vi "BG Selection List get.vi"(0 "QD Launch VI Ref":refnum<vi>, 11 "error in (no error)":errorcluster) -> (4 "QD Launch VI Ref out":refnum<vi>, 8 "Selection List[]":refnum<vi>[](array[refnum]), 15 "error out":errorcluster)   [LabVIEW 2020, in "ColourUpStructures.lvlib"]
doc: "From QuickDrop Lunched VI reference extract All Selected GObject on Block Diagram"
uses:
  ColourUpStructures.lvlib
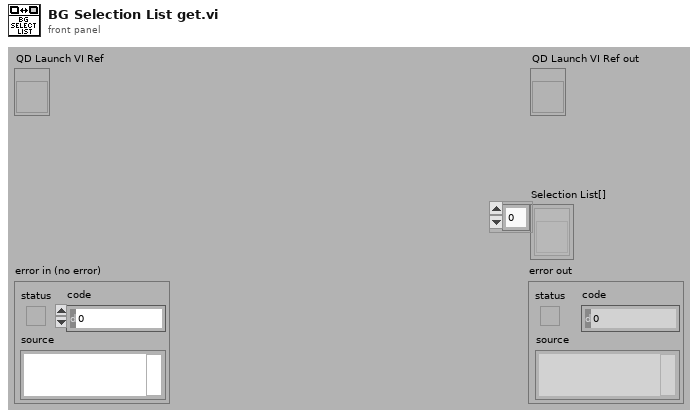
[diagram p1: front panel]
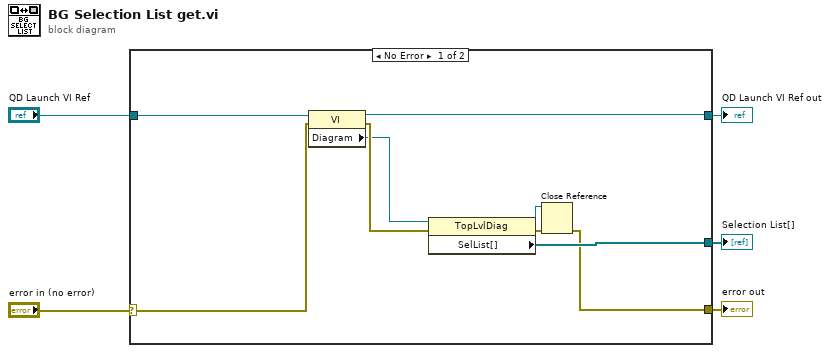
[diagram p0: block diagram]
diagram:
  n1 = case shown="No Error" "error in (no error)" {
    selector: "error in (no error)" -> [w9 w16]
    tunnel: "QD Launch VI Ref" -> [w14 w15]
    tunnel: [w7 w16] -> w4
    tunnel: [w8 _] -> w2
    tunnel: [w6 w15] -> w1
    frame No Error {
      n2 = property class="VI"(reference=w14, error in=w9) -> (reference out=w6:refnum<vi>, error out=w11:errorcluster, "Diagram"=w10:refnum<vi>)
      n3 = property class="TopLvlDiag"(reference=w10, error in=w11) -> (reference out=w13:refnum<vi>, error out=w12:errorcluster, "SelList[]"=w8:refnum<vi>[])
      n4 = Close Reference(reference=w13, error in (no error)=w12) -> (error out=w7:errorcluster)
    }
    frame Error {
    }
  }
  "Selection List[]" <- w2
  "error out" <- w4
  "QD Launch VI Ref out" <- w1
